vi "GetMsgData.vi"(8 "error in (no error)":errorcluster, 11 "UpstreamMsgParent in":refnum<class "UpstreamMsgParent.lvclass">) -> (0 "error out":errorcluster, 2 "MsgData":variant, 3 "UpstreamMsgParent out":refnum<class "UpstreamMsgParent.lvclass">)   [LabVIEW 2020, in "UpstreamMsg.lvlib" / "UpstreamMsgParent.lvclass"]
doc: "This is used in the scripting to create the go, it provides the datatype"
uses:
  UpstreamMsgParent/UpstreamMsgParent.lvclass
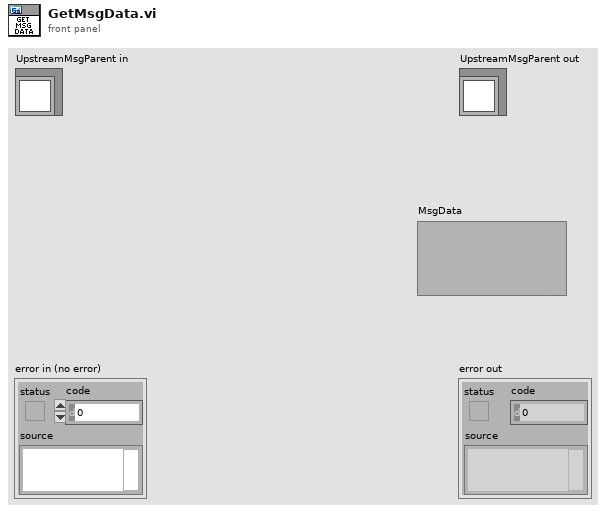
[diagram p1: front panel]
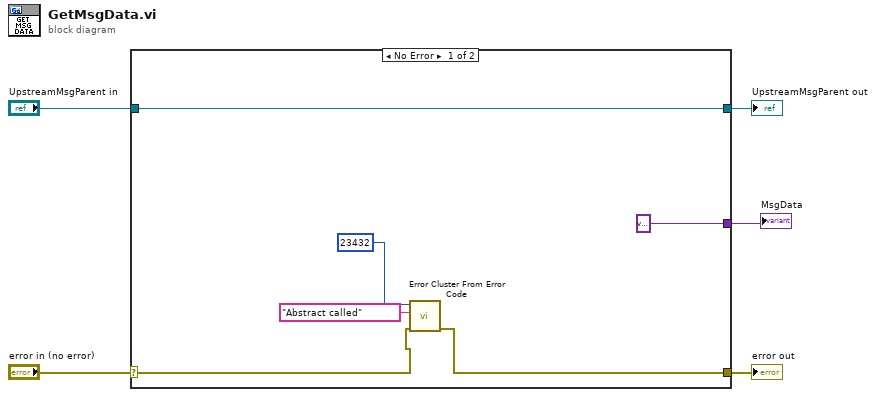
[diagram p0: block diagram]
diagram:
  n1 = case shown="No Error" "error in (no error)" {
    selector: "error in (no error)" -> [w8 w13]
    tunnel: [w7 w13] -> w4
    tunnel: [w11 w12] -> w2
    tunnel: "UpstreamMsgParent in" -> [w11 w12]
    tunnel: [variant ("MsgData") _] -> w1
    frame No Error {
      n2 = call <vilib>:"Error Cluster From Error Code.vi"("error in (no error)"=w8, "error message (\"\")"="Abstract called" ("error message (\"\")"), "error code (0)"=23432) -> ("error out"=w7:errorcluster)  [unwired: 6 in]
    }
    frame Error {
    }
  }
  "error out" <- w4
  "UpstreamMsgParent out" <- w2
  "MsgData" <- w1
